vi "Read Temp.vi"(8 "error in (no error)":errorcluster, 10 "Temp Chan":string, 11 "IP Address in":string) -> (0 "error out":errorcluster, 3 "Temperature":dbl)   [LabVIEW 2024]
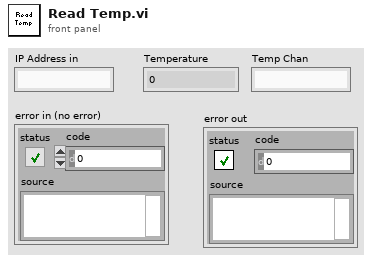
[diagram p1: front panel]
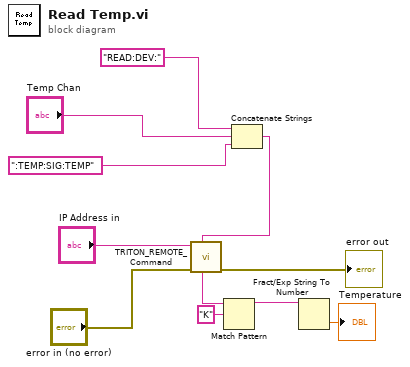
[diagram p0: block diagram]
diagram:
  n1 = Concatenate Strings("READ:DEV:" ("string"), "Temp Chan", ":TEMP:SIG:TEMP" ("Command to send")) -> (w1:string)
  n2 = call "TRITON_REMOTE_Command.vi"("Command to send"=w1, "error in (no error)"="error in (no error)", "IP Address"="IP Address in") -> ("error out"=→"error out":errorcluster, "Trimmed String"=w10:string)  [unwired: 6 in, 1 out]
  n3 = Match Pattern(string=w10, regular expression="K") -> (before substring=w6:string)  [unwired: 1 in, 3 out]
  n4 = Fract/Exp String To Number(string=w6) -> (number=→"Temperature":dbl)  [unwired: 3 in, 1 out]
